vi "facade.vi"(0 "Data In":T10 caption="Données en entrée" {"slot#" max=4095; "DAC"."DAC offset" min=-1 max=0.5; "DAC"."FastChanNum" max=15 step=1}, 2 "Display State In":T8 caption="État d'affichage en entrée", 3 "Container State":T9 caption="État du conteneur") -> (6 "Data Out":T10 caption="Données en sortie" {"slot#" max=4095; "DAC"."DAC offset" min=-1 max=0.5; "DAC"."FastChanNum" max=15 step=1}, 7 "Display State Out":T8 caption="État d'affichage en sortie", 8 "Action":T7)   [LabVIEW 2013, in "slot.xctl"]
uses:
  slot.xctl
  data.ctl
  slot-use.ctl
  triggers.ctl
  DAC.ctl
  DAC_fastseq-offset.ctl
  timing.ctl
  jump.ctl
  <vilib>/_xctls/Container State.ctl
  state.ctl
  <vilib>/_xctls/Action.ctl
  <vilib>/_xctls/XControlSupport.lvlib
panel:
  in  "slot#":T1 max=4095
  in  "DAC":T2 {"DAC offset" min=-1 max=0.5; "FastChanNum" max=15 step=1}
  in  "timing":T4
  in  "Triggers":T5
  in  "use":T6
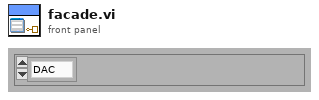
[diagram p1: front panel]
types:
  T1 = typedef "jump.ctl" = u16
  T2 = typedef "DAC.ctl" = cluster{"FastChanNum":u8, "DAC offset":T3}
  T3 = typedef "DAC_fastseq-offset.ctl" = sgl
  T4 = typedef "timing.ctl" = sgl
  T5 = typedef "triggers.ctl" = cluster{"triggers":cluster{"1":bool, "2":bool, "3":bool, "4":bool}, "stop":bool}
  T6 = typedef "slot-use.ctl" = enum8{"DAC", "timing", "triggers", "jump"}
  T7 = typedef "XControlSupport.lvlib/Action.ctl" = cluster{"Data Changed?":bool, "State Changed?":bool, "Action Name":string}
  T8 = typedef "slot.xctl/state.ctl" = cluster{"use":T6}
  T9 = typedef "XControlSupport.lvlib/Container State.ctl" = cluster{"Indicator?":bool, "Run Mode?":bool, " Refnum":refnum<vi>}
  T10 = typedef "slot.xctl/data.ctl" = cluster{"use":T6, "Triggers":T5, "DAC":T2, "timing":T4, "slot#":T1}
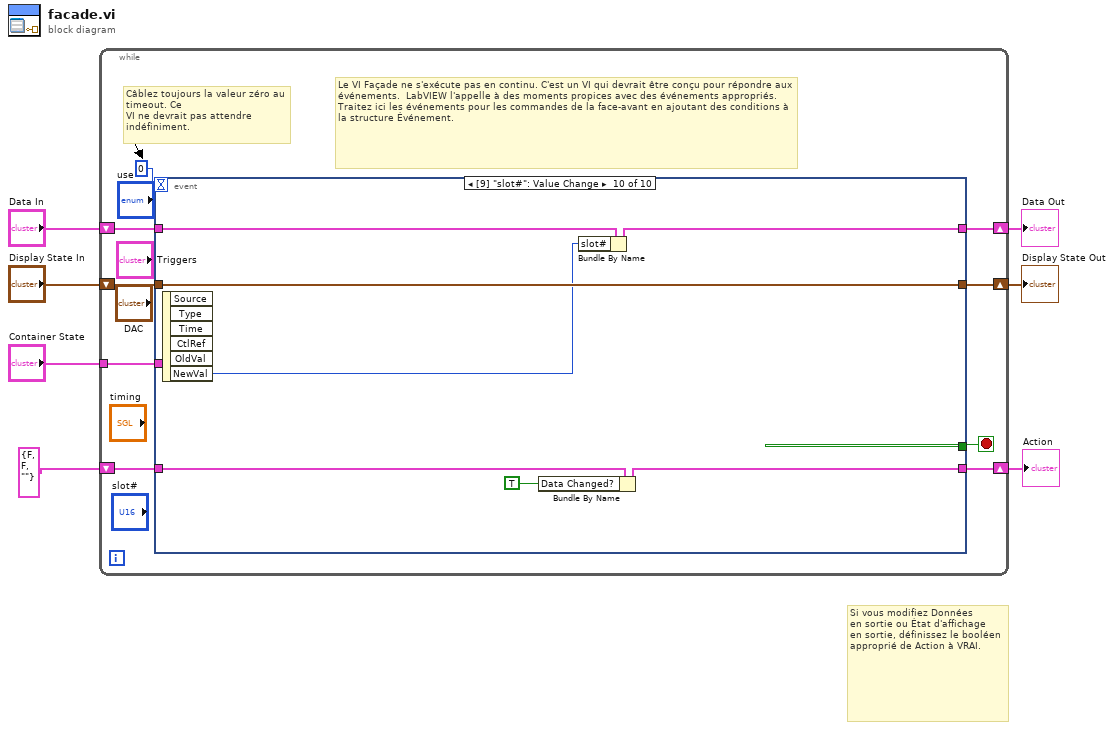
[diagram p0: block diagram]
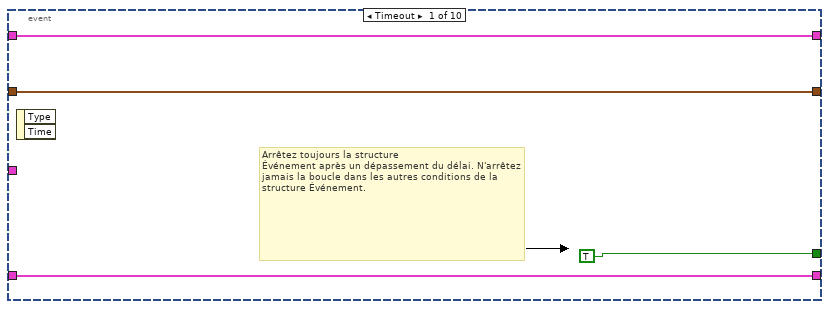
[diagram p2: hidden frame]
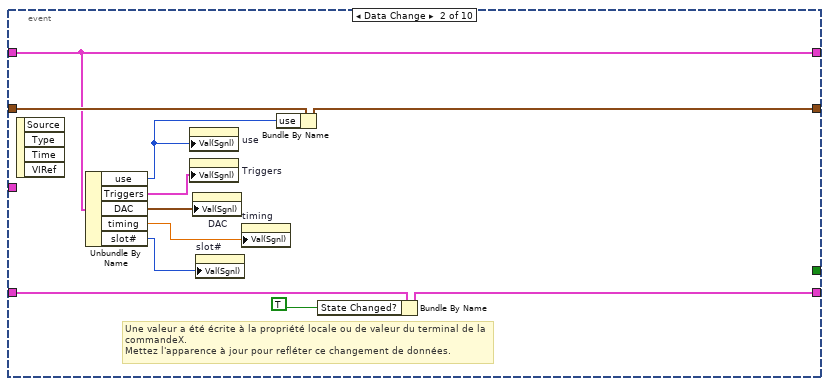
[diagram p3: hidden frame]
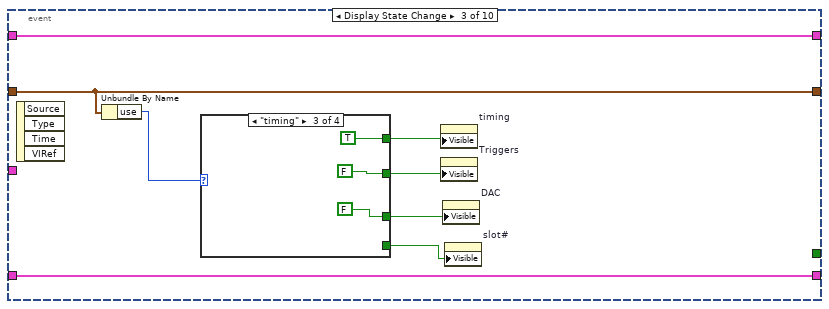
[diagram p4: hidden frame]
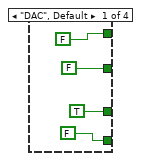
[diagram p5: hidden frame]
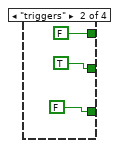
[diagram p6: hidden frame]
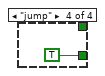
[diagram p7: hidden frame]
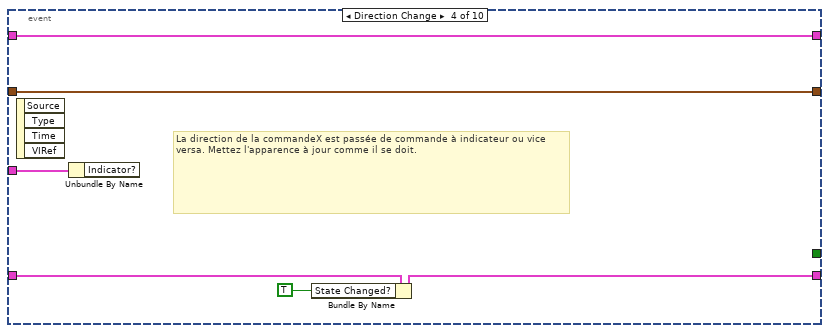
[diagram p8: hidden frame]
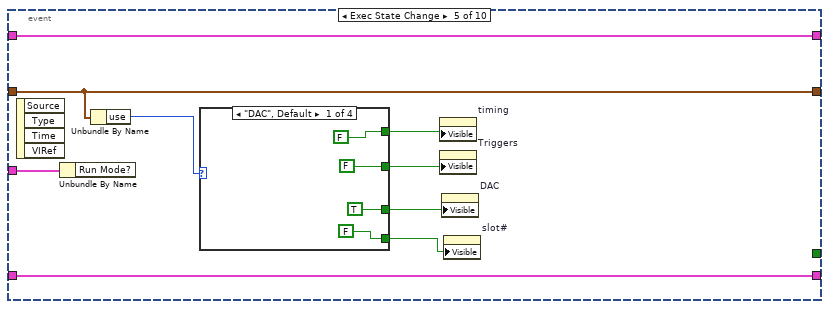
[diagram p9: hidden frame]
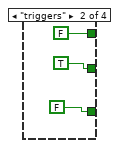
[diagram p10: hidden frame]
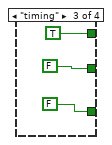
[diagram p11: hidden frame]
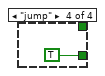
[diagram p12: hidden frame]
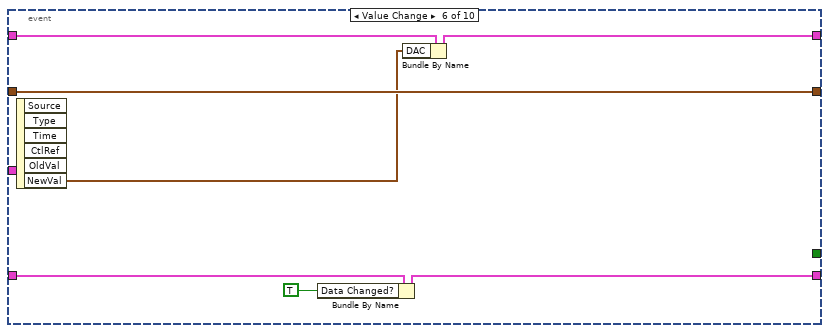
[diagram p13: hidden frame]
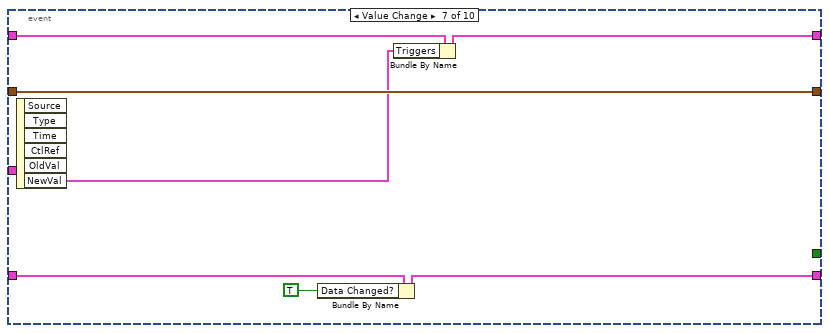
[diagram p14: hidden frame]
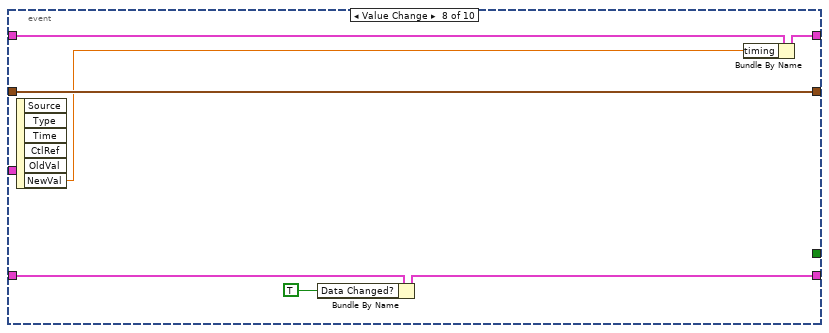
[diagram p15: hidden frame]
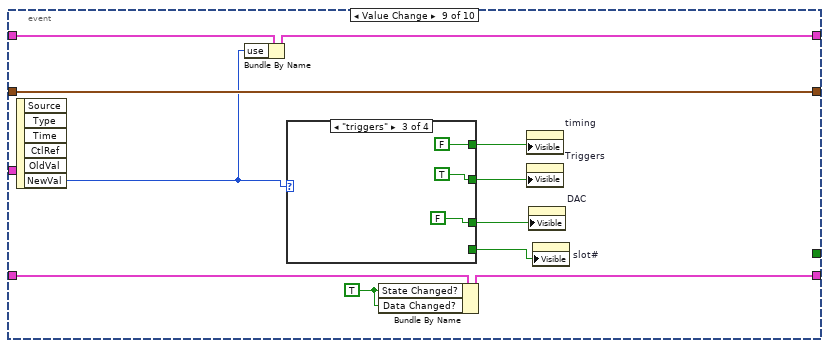
[diagram p16: hidden frame]
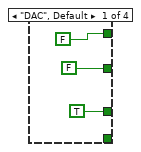
[diagram p17: hidden frame]
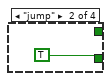
[diagram p18: hidden frame]
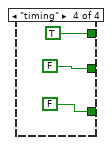
[diagram p19: hidden frame]
diagram:
  # "Si vous modifiez Données\nen sortie ou État d'affichage\nen sortie, définissez le booléen\napproprié de Action à VRAI."
  n1 = while {
    shift-right: [w15] -> w4
    shift-left: "Display State In" -> [w16]
    tunnel: "Container State" -> [w12]
    shift-right: [w10] -> w7
    shift-left: "Data In" -> [w11]
    shift-right: [w8] -> w2
    shift-left: T7 {"Data Changed?"=FALSE, "State Changed?"=FALSE, "Action Name"=""} ("Action") -> [w9]
    stop <- w14 stop-if-true
    # "Le VI Façade ne s'exécute pas en continu. C'est un VI qui devrait être conçu pour répondre aux événements.  LabVIEW l'appelle à des moments propices avec des événements appropriés. Traitez ici les événements pour les commandes de la face-avant en ajoutant des conditions à la structure Événement."
    # "Câblez toujours la valeur zéro au timeout. Ce\nVI ne devrait pas attendre indéfiniment."
    n2 = event shown="[9] \"slot#\": Value Change" {
      selector: _ -> [_ _ _ _ _ _ _ _ _ _]
      dyn-events: _ -> [_ _ _ _ _ _ _ _ _ _]
      timeout: 0 -> [_ _ _ _ _ _ _ _ _ _]
      tunnel: w16 -> [w18 w31 w33 w55 w59 w83 w90 w97 w102 w122]
      tunnel: [w18 w29 w33 w55 w59 w83 w90 w97 w102 w122] -> w15
      tunnel: [TRUE _ _ _ _ _ _ _ _ _] -> w14
      tunnel: w12 -> [_ _ _ w56 w65 _ _ _ _ _]
      tunnel: w11 -> [w17 w28 w39 w54 w64 w82 w89 w96 w106 w121]
      tunnel: [w17 w28 w39 w54 w64 w81 w88 w95 w101 w120] -> w10
      tunnel: [w19 w22 w38 w52 w63 w78 w86 w93 w107 w124] -> w8
      tunnel: w9 -> [w19 w30 w38 w53 w63 w79 w87 w94 w108 w125]
      event Timeout {
        # "Arrêtez toujours la structure\nÉvénement après un dépassement du délai. N'arrêtez jamais la boucle dans les autres conditions de la structure Événement."
        n3 = event-data() -> ()  [unwired: 3 out]
      }
      event Data Change {
        # "Une valeur a été écrite à la propriété locale ou de valeur du terminal de la commandeX.\nMettez l'apparence à jour pour refléter ce changement de données."
        n4 = event-data() -> ()  [unwired: 5 out]
        n5 = Unbundle By Name(w28) -> ("use"=w23:T6, "Triggers"=w27:T5, "DAC"=w26:T2, "timing"=w25:T4, "slot#"=w24:T1)
        n6 = property on="use" class="Enum (strict)"("Val(Sgnl)"=w23) -> ()  [unwired: 2 in, 2 out]
        n7 = property on="Triggers" class="Clust (strict)"("Val(Sgnl)"=w27) -> ()  [unwired: 2 in, 2 out]
        n8 = property on="DAC" class="Clust (strict)"("Val(Sgnl)"=w26) -> ()  [unwired: 2 in, 2 out]
        n9 = property on="slot#" class="DigNum (strict)"("Val(Sgnl)"=w24) -> ()  [unwired: 2 in, 2 out]
        n10 = property on="timing" class="DigNum (strict)"("Val(Sgnl)"=w25) -> ()  [unwired: 2 in, 2 out]
        n11 = Bundle By Name(cluster=w31, "use"=w23) -> (w29:T8)
        n12 = Bundle By Name(cluster=w30, "State Changed?"=TRUE) -> (w22:T7)
      }
      event Display State Change {
        n13 = event-data() -> ()  [unwired: 5 out]
        n14 = Unbundle By Name(w33) -> ("use"=w32:T6)
        n15 = case shown="\"timing\"" w32 {
          tunnel: [FALSE ("Visible") FALSE ("Visible") TRUE ("Visible") _] -> w37
          tunnel: [FALSE ("Visible") TRUE ("Visible") FALSE ("Visible") _] -> w36
          tunnel: [TRUE ("Visible") FALSE ("Visible") FALSE ("Visible") _] -> w35
          tunnel: [FALSE ("Visible") _ _ TRUE ("Visible")] -> w34
          frame "DAC", Default {
          }
          frame "triggers" {
          }
          frame "timing" {
          }
          frame "jump" {
          }
        }
        n16 = property on="timing" class="DigNum (strict)"("Visible"=w37) -> ()  [unwired: 2 in, 2 out]
        n17 = property on="Triggers" class="Clust (strict)"("Visible"=w36) -> ()  [unwired: 2 in, 2 out]
        n18 = property on="DAC" class="Clust (strict)"("Visible"=w35) -> ()  [unwired: 2 in, 2 out]
        n19 = property on="slot#" class="DigNum (strict)"("Visible"=w34) -> ()  [unwired: 2 in, 2 out]
      }
      event Direction Change {
        # "La direction de la commandeX est passée de commande à indicateur ou vice versa. Mettez l'apparence à jour comme il se doit."
        n20 = event-data() -> ()  [unwired: 5 out]
        n21 = Unbundle By Name(w56) -> ()  [unwired: 1 out]
        n22 = Bundle By Name(cluster=w53, "State Changed?"=TRUE) -> (w52:T7)
      }
      event Exec State Change {
        n23 = event-data() -> ()  [unwired: 5 out]
        n24 = Unbundle By Name(w65) -> ()  [unwired: 1 out]
        n25 = Unbundle By Name(w59) -> ("use"=w58:T6)
        n26 = case shown="\"DAC\", Default" w58 {
          tunnel: [FALSE ("Visible") FALSE ("Visible") TRUE ("Visible") _] -> w62
          tunnel: [FALSE ("Visible") TRUE ("Visible") FALSE ("Visible") _] -> w61
          tunnel: [TRUE ("Visible") FALSE ("Visible") FALSE ("Visible") _] -> w60
          tunnel: [FALSE ("Visible") _ _ TRUE ("Visible")] -> w57
          frame "DAC", Default {
          }
          frame "triggers" {
          }
          frame "timing" {
          }
          frame "jump" {
          }
        }
        n27 = property on="timing" class="DigNum (strict)"("Visible"=w62) -> ()  [unwired: 2 in, 2 out]
        n28 = property on="Triggers" class="Clust (strict)"("Visible"=w61) -> ()  [unwired: 2 in, 2 out]
        n29 = property on="DAC" class="Clust (strict)"("Visible"=w60) -> ()  [unwired: 2 in, 2 out]
        n30 = property on="slot#" class="DigNum (strict)"("Visible"=w57) -> ()  [unwired: 2 in, 2 out]
      }
      event Value Change {
        n31 = event-data() -> ("NewVal"=w80:T2)  [unwired: 6 out]
        n32 = Bundle By Name(cluster=w79, "Data Changed?"=TRUE) -> (w78:T7)
        n33 = Bundle By Name(cluster=w82, "DAC"=w80) -> (w81:T10)
      }
      event Value Change {
        n34 = event-data() -> ("NewVal"=w84:T5)  [unwired: 6 out]
        n35 = Bundle By Name(cluster=w87, "Data Changed?"=TRUE) -> (w86:T7)
        n36 = Bundle By Name(cluster=w89, "Triggers"=w84) -> (w88:T10)
      }
      event Value Change {
        n37 = event-data() -> ("NewVal"=w91:T4)  [unwired: 6 out]
        n38 = Bundle By Name(cluster=w94, "Data Changed?"=TRUE) -> (w93:T7)
        n39 = Bundle By Name(cluster=w96, "timing"=w91) -> (w95:T10)
      }
      event Value Change {
        w99 = TRUE ("State Changed?")
        n40 = event-data() -> ("NewVal"=w100:T6)  [unwired: 6 out]
        n41 = Bundle By Name(cluster=w106, "use"=w100) -> (w101:T10)
        n42 = case shown="\"triggers\"" w100 {
          tunnel: [FALSE ("Visible") _ FALSE ("Visible") TRUE ("Visible")] -> w105
          tunnel: [FALSE ("Visible") _ TRUE ("Visible") FALSE ("Visible")] -> w104
          tunnel: [TRUE ("Visible") _ FALSE ("Visible") FALSE ("Visible")] -> w103
          tunnel: [_ TRUE ("State Changed?") _ _] -> w98
          frame "DAC", Default {
          }
          frame "jump" {
          }
          frame "triggers" {
          }
          frame "timing" {
          }
        }
        n43 = Bundle By Name(cluster=w108, "State Changed?"=w99, "Data Changed?"=w99) -> (w107:T7)
        n44 = property on="timing" class="DigNum (strict)"("Visible"=w105) -> ()  [unwired: 2 in, 2 out]
        n45 = property on="Triggers" class="Clust (strict)"("Visible"=w104) -> ()  [unwired: 2 in, 2 out]
        n46 = property on="DAC" class="Clust (strict)"("Visible"=w103) -> ()  [unwired: 2 in, 2 out]
        n47 = property on="slot#" class="DigNum (strict)"("Visible"=w98) -> ()  [unwired: 2 in, 2 out]
      }
      event Value Change {
        n48 = event-data() -> ("NewVal"=w119:T1)  [unwired: 6 out]
        n49 = Bundle By Name(cluster=w125, "Data Changed?"=TRUE) -> (w124:T7)
        n50 = Bundle By Name(cluster=w121, "slot#"=w119) -> (w120:T10)
      }
    }
  }
  "Display State Out" <- w4
  "Data Out" <- w7
  "Action" <- w2
